vi "FPGA Draw background.vi"(10 "Row":u16, 11 "Col":u16) -> ()   [LabVIEW 2019]
uses:
  <vilib>/rvi/Memory/Memory_Emulation/nirvimemoryFastEmulation.vi
  <vilib>/rvi/Memory/Memory_Emulation/nirvimemoryEmulation.vi
  <vilib>/rvi/Emulation/niFpgaEmulationIsFPGAContextNoSignature.vi
  <vilib>/rvi/DataTransferAndStorage/Container/Common/niFpgaContainerGetUniqueNameForEmu.vi
  <vilib>/rvi/Emulation/niFpgaProcessEmulError.vi
  <vilib>/rvi/Emulation/niFpgaSctlEmulationGetInTimedLoop.vi
  <vilib>/rvi/errors/nirviReportUnexpectedCaseInternalError (U32).vi
  <vilib>/rvi/DataTransferAndStorage/Container/XNode/niFpgaContainer.xnode
panel:
  # "y"
  # "x"
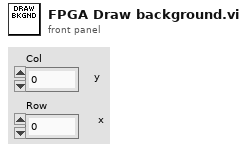
[diagram p1: front panel]
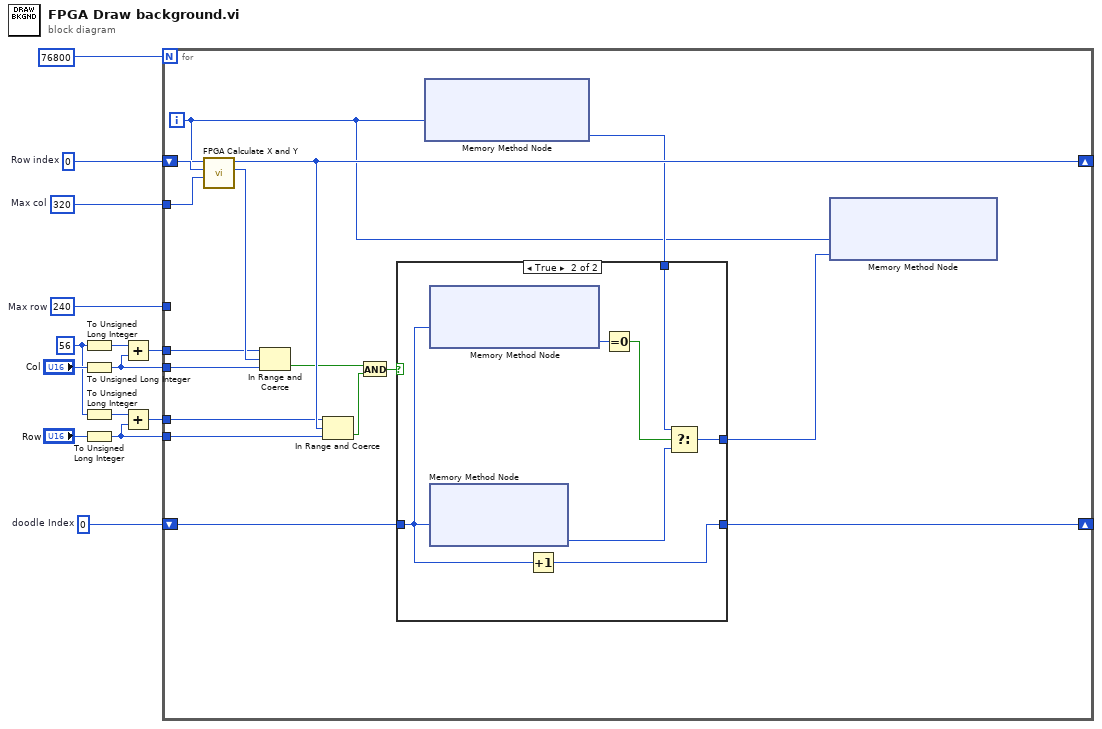
[diagram p0: block diagram]
diagram:
  w1 = u32 0  # doodle Index
  w11 = u32 0  # Row index
  w12 = i16 240  # Max row
  w13 = i16 320  # Max col
  w3 = i16 56
  n1 = To Unsigned Long Integer(number=w3) -> (unsigned 32bit integer=w7:u32)
  n2 = To Unsigned Long Integer(number="Col") -> (unsigned 32bit integer=w8:u32)
  n3 = To Unsigned Long Integer(number=w3) -> (unsigned 32bit integer=w6:u32)
  n4 = To Unsigned Long Integer(number="Row") -> (unsigned 32bit integer=w4:u32)
  n5 = Add(x=w7, y=w8) -> (x+y=w9:u32)
  n6 = Add(x=w6, y=w4) -> (x+y=w2:u32)
  n7 = for {
    N: 76800 -> [_]
    tunnel: w8 -> [w26]
    tunnel: w13 -> [w29]
    tunnel: w12 -> [_]
    shift-right: [w25] -> _
    shift-left: w11 -> [w30]
    tunnel: w9 -> [w27]
    tunnel: w4 -> [w23]
    tunnel: w2 -> [w24]
    shift-right: [w18] -> _
    shift-left: w1 -> [w19]
    i -> [w16]
    n8 = call "FPGA Calculate X and Y.vi"("Max col"=w29, "Row index in"=w30, "Current Interation"=w16) -> ("Col index out"=w28:u32, "Row index out"=w25:u32)  [unwired: 7 in]
    n9 = In Range and Coerce(upper limit=w27, x=w28, lower limit=w26) -> (In Range?=w21:bool)  [unwired: 1 out]
    n10 = In Range and Coerce(upper limit=w24, x=w25, lower limit=w23) -> (In Range?=w22:bool)  [unwired: 1 out]
    n11 = And(x=w21, y=w22) -> (x .and. y?=w20:bool)
    n12 = xnode ("Memory Method Node")("Address"=w16) -> ("Data"=w17:u16)  [unwired: 1 in, 1 out]
    n13 = case shown="True" w20 {
      tunnel: w19 -> [w32 w33]
      tunnel: [w32 w39] -> w18
      tunnel: w17 -> [w31 w35]
      tunnel: [w31 w34] -> w15
      frame False {
      }
      frame True {
        n14 = xnode ("Memory Method Node")("Address"=w33) -> ("Data"=w38:u8)  [unwired: 1 in, 1 out]
        n15 = xnode ("Memory Method Node")("Address"=w33) -> ("Data"=w36:u16)  [unwired: 1 in, 1 out]
        n16 = Increment(x=w33) -> (x+1=w39:u32)
        n17 = Equal To 0?(x=w38) -> (x = 0?=w37:bool)
        n18 = Select(t=w35, s=w37, f=w36) -> (s? t:f=w34:u16)
      }
    }
    n19 = xnode ("Memory Method Node")("Address"=w16, "Data"=w15) -> ()  [unwired: 1 in, 1 out]
  }
